vi "Read Music Folder Path.vi"(8 "error in (no error)":errorcluster) -> (0 "error out":errorcluster, 3 "Music Folder Path":path)   [LabVIEW 2015, in "App Config.lvlib"]
uses:
  App Config.lvlib
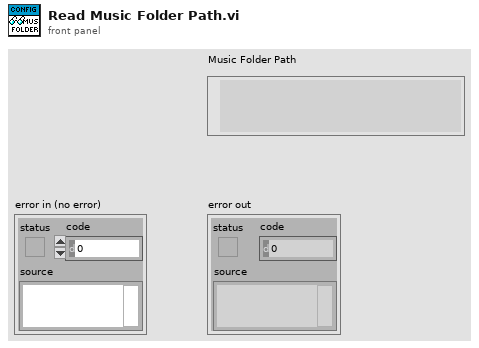
[diagram p1: front panel]
types:
  T1 = typedef "App Config.lvlib/App Config Data.ctl" = cluster{"Music Folder Path":path, "Temp Images Path":path}
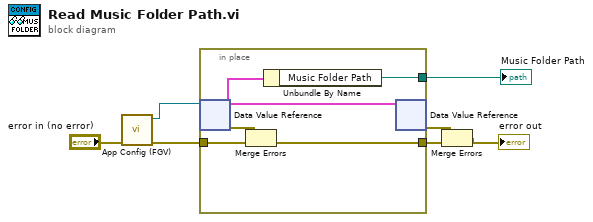
[diagram p0: block diagram]
diagram:
  n1 = call "App Config (FGV).vi"("error in (no error)"="error in (no error)") -> ("error out"=w6:errorcluster, "DVR Out"=w5:refnum<data-value>)  [unwired: 9 in]
  n2 = in-place {
    in-place-border: w6 -> [w12]
    in-place-border: [w10] -> w4
    in-place-border: [w9] -> w2
    n3 = in-place-dvr #1(w5) -> (w8:T1, w11:errorcluster)
    n4 = Merge Errors(w11, w12) -> (w9:errorcluster)
    n5 = Unbundle By Name(w8) -> ("Music Folder Path"=w10:path)
    n6 = in-place-dvr #1(w8) -> (w1:errorcluster)  [unwired: 1 out]
  }
  "Music Folder Path" <- w4
  n7 = Merge Errors(w1, w2) -> (→"error out":errorcluster)
